vi "Write_parameter.vi"(8 "error in (no error)":errorcluster caption="entrée d'erreur (pas d'erreur)", 10 "Parameter":string, 11 "Class DIO en entrée":refnum<class "Class Instrument Log_File.lvclass">) -> (0 "error out":errorcluster caption="sortie d'erreur", 3 "Class DIO en Sortie":refnum<class "Class Instrument Log_File.lvclass">)   [LabVIEW 2020, in "Library Instrument & Equipement.lvlib" / "Library Instruments.lvlib" / "Class Instrument Log_File.lvclass"]
uses:
  Class Instrument Log_File.lvclass
  Commun VI/TypeDef/Commande Test/Commande Data Test.ctl
  Commun VI/TypeDef/Commande Test/Commande Value Type.ctl
  Commun VI/TypeDef/Commande Test/Commande Type Test.ctl
  Log File/Class Log_File Altyor/Class Log_File Altyor.lvclass
  JSON API/JSON Value/Set from JSON string.vi
  Instrument (Default)/Class Instrument (Default).lvclass
  JSON API/JSON Value/JSON Value.lvclass
  Class Instrument Log_File.lvclass/Class Instrument Log_File.ctl
  JSON API/Variant JSON/Variant JSON.lvlib
  JSON API/Get Polymorphic/JSON GetSet.lvlib
  Commun VI/Library Commun.lvlib
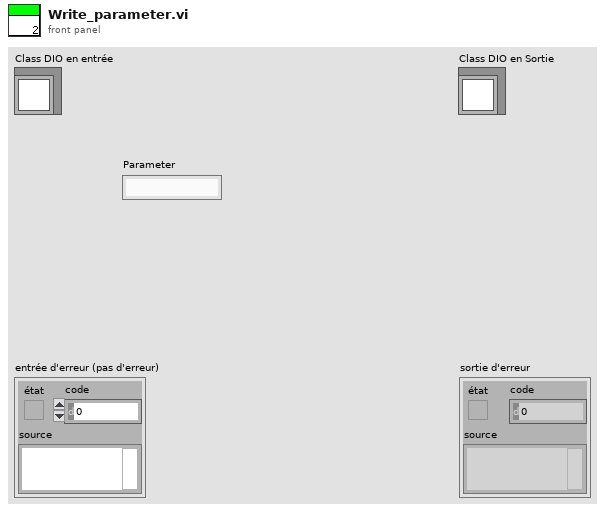
[diagram p1: front panel]
types:
  T1 = cluster{"Path_Log_File":path, "Delimit":string, "File For Save":refnum<queue>, "Event Error":refnum<user-event>, "Class Log_File":refnum<class "Class Log_File Altyor.lvclass">}
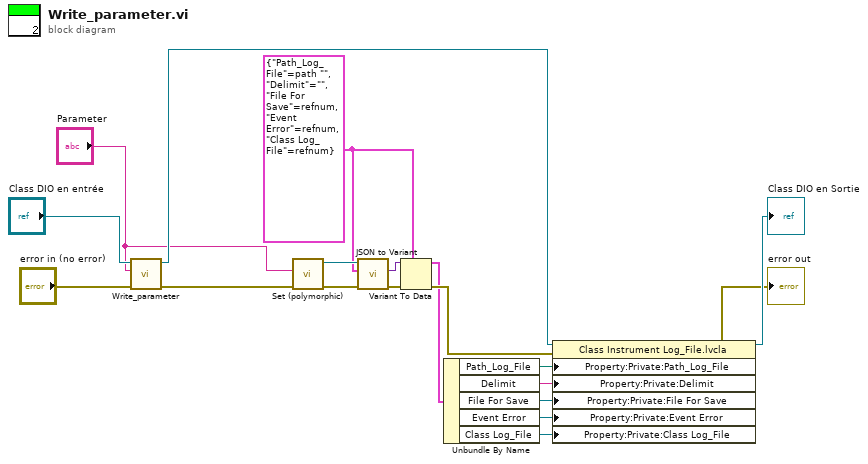
[diagram p0: block diagram]
diagram:
  w1 = T1 {"Path_Log_File"=path "", "Delimit"="", "File For Save"=refnum, "Event Error"=refnum, "Class Log_File"=refnum} ("Parameter")
  n1 = call-parent "Write_parameter.vi"("error in (no error)"="error in (no error)", "Parameter"="Parameter", "Class Instrument (Default) en entrée"="Class DIO en entrée") -> ("error out"=w8:errorcluster, "Class Instrument (Default) en sortie"=w6:refnum<class "Class Instrument Log_File.lvclass">)  [unwired: 7 in]
  n2 = call-poly "Set (polymorphic).vi"("error in (no error)"=w8, "JSON stream"="Parameter") -> ("error out"=w17:errorcluster, "JSON Value out"=w19:refnum<class "JSON Value.lvclass">)  [unwired: 7 in, 1 out]
  n3 = call "JSON to Variant.vi"("error in (no error)"=w17, "Variant (Data Type)"=w1, "JSON Value"=w19) -> ("error out"=w18:errorcluster, "Variant out"=w16:variant)  [unwired: 7 in]
  n4 = Variant To Data(error in=w18, type=w1, Variant=w16) -> (data=w11:T1, error out=w12:errorcluster)
  n5 = Unbundle By Name(w11) -> ("Path_Log_File"=w9:path, "Delimit"=w10:string, "File For Save"=w4:refnum<queue>, "Event Error"=w3:refnum<user-event>, "Class Log_File"=w2:refnum<class "Class Log_File Altyor.lvclass">)
  n6 = property class="Class Instrument Log_File.lvcla"(reference=w6, error in=w12, "Property:Private:Path_Log_File"=w9, "Property:Private:Delimit"=w10, "Property:Private:File For Save"=w4, "Property:Private:Event Error"=w3, "Property:Private:Class Log_File"=w2) -> (reference out=→"Class DIO en Sortie":refnum<class "Class Instrument Log_File.lvclass">, error out=→"error out":errorcluster)
